vi "Launch Sample Line.vi"(8 "error in (no error)":errorcluster, 11 "cRIO-CO2 in":refnum<class "cRIO-CO2.lvclass">) -> (0 "error out":errorcluster, 3 "cRIO-CO2 out":refnum<class "cRIO-CO2.lvclass">)   [LabVIEW 2015, in "cRIO-Carbondioxide.lvlib" / "cRIO-CO2.lvlib" / "cRIO-CO2.lvclass"]
uses:
  cRIO-CO2.lvclass
  Sample Line/Sample Line.lvclass
  CO2 Actor/CO2 Actor.lvclass
  <vilib>/ActorFramework/Actor/Actor.lvclass
  cRIO-CO2.lvclass/cRIO-CO2.ctl
  cRIO-CO2 Messages/Log Message Msg/Log Message Msg.lvclass/Log Message Msg.ctl
  <vilib>/ActorFramework/Message Enqueuer/Message Enqueuer.lvclass/Message Enqueuer.ctl
  <vilib>/ActorFramework/Message Enqueuer/Enqueue.vi
  <vilib>/ActorFramework/Message Priority Queue/Priority Enqueue.vi
  <vilib>/ActorFramework/Message Enqueuer/Message Enqueuer.lvclass
  cRIO-CO2 Messages/Log Message Msg/Log Message Msg.lvclass
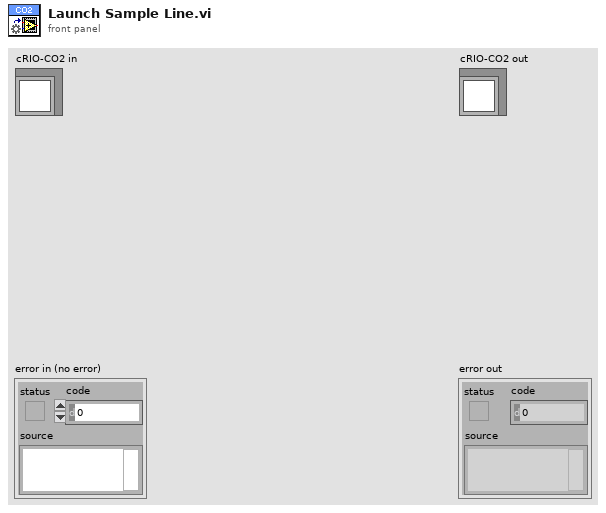
[diagram p1: front panel]
types:
  T1 = typedef "Dedicated Enqueuers.ctl" = cluster{"Freezers":cluster{"Syringe":refnum<class "Message Enqueuer.lvclass">, "Tank 1":refnum<class "Message Enqueuer.lvclass">, "Tank 2":refnum<class "Message Enqueuer.lvclass">, "Tank 3":refnum<class "Message Enqueuer.lvclass">, "Tank 4":refnum<class "Message Enqueuer.lvclass">}, "Heaters":cluster{"Syringe":refnum<class "Message Enqueuer.lvclass">, "Piston":refnum<class "Message Enqueuer.lvclass">}, "Blowers":cluster{"Tank 1":refnum<class "Message Enqueuer.lvclass">, "Tank 2":refnum<class "Message Enqueuer.lvclass">, "Tank 3":refnum<class "Message Enqueuer.lvclass">, "Tank 4":refnum<class "Message Enqueuer.lvclass">, "Syringe":refnum<class "Message Enqueuer.lvclass">}, "Sample Line":refnum<class "Message Enqueuer.lvclass">, "Storage Line":refnum<class "Message Enqueuer.lvclass">, "Transfer Line":refnum<class "Message Enqueuer.lvclass">, "Syringe Stepper":refnum<class "Message Enqueuer.lvclass">, "Syringe Line":refnum<class "Message Enqueuer.lvclass">, "Capillary Line":refnum<class "Message Enqueuer.lvclass">, "Preparation Line":refnum<class "Message Enqueuer.lvclass">, "Turbo":refnum<class "Message Enqueuer.lvclass">, "Vacuum":refnum<class "Message Enqueuer.lvclass">, "He Line":refnum<class "Message Enqueuer.lvclass">, "Cylinder":refnum<class "Message Enqueuer.lvclass">}
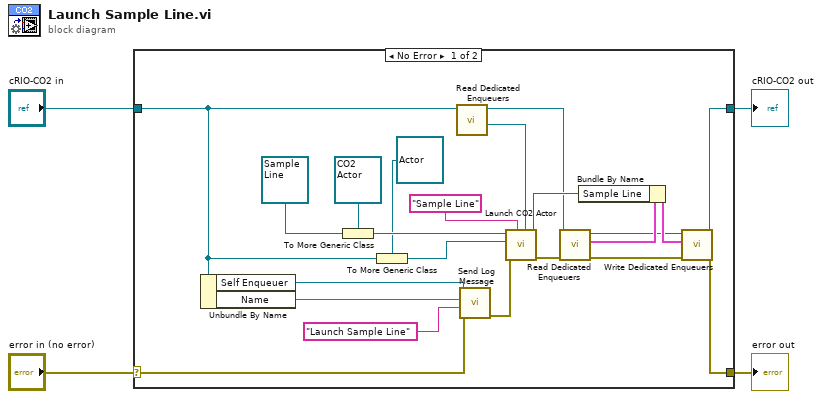
[diagram p0: block diagram]
diagram:
  n1 = case shown="No Error" "error in (no error)" {
    selector: "error in (no error)" -> [w24 w28]
    tunnel: [w14 w28] -> w3
    tunnel: [w12 w27] -> w1
    tunnel: "cRIO-CO2 in" -> [w11 w27]
    frame No Error {
      n2 = Unbundle By Name(w11) -> ("Self Enqueuer"=w7:refnum<class "Message Enqueuer.lvclass">, "Name"=w21:string)
      n3 = To More Generic Class(target class=refnum<class "CO2 Actor.lvclass"> refnum ("CO2 Actor in"), reference=refnum<class "Sample Line.lvclass"> refnum ("Sample Line.lvclass")) -> (generic class reference=w25:refnum<class "CO2 Actor.lvclass">)
      n4 = To More Generic Class(target class=refnum<class "Actor.lvclass"> refnum ("Caller Actor in"), reference=w11) -> (generic class reference=w8:refnum<class "Actor.lvclass">)
      n5 = call "Read Dedicated Enqueuers.vi"("cRIO-CO2 in"=w11) -> ("Qs.DedicatedEnQrs"=w5:refnum<queue>, "cRIO-CO2 out"=w6:refnum<class "cRIO-CO2.lvclass">)  [unwired: 7 in, 2 out]
      n6 = call "Send Log Message.vi"("error in (no error)"=w24, "String"="Launch Sample Line", "Source Name"=w21, "Message Enqueuer"=w7) -> ("error out"=w23:errorcluster)  [unwired: 6 in, 1 out]
      n7 = call "Launch CO2 Actor.vi"("DedicatedEnQrs"=w5, "Name"="Sample Line", "error in (no error)"=w23, "Caller Actor in"=w8, "CO2 Actor in"=w25) -> ("error out"=w15:errorcluster, "Caller-To-Actor Enqueuer"=w19:refnum<class "Message Enqueuer.lvclass">)  [unwired: 5 in]
      n8 = call "Read Dedicated Enqueuers.vi"("error in (no error)"=w15, "cRIO-CO2 in"=w6) -> ("error out"=w16:errorcluster, "Dedicated Enqueuers"=w18:T1, "cRIO-CO2 out"=w13:refnum<class "cRIO-CO2.lvclass">)  [unwired: 6 in, 1 out]
      n9 = Bundle By Name(cluster=w18, "Sample Line"=w19) -> (w17:T1)
      n10 = call "Write Dedicated Enqueuers.vi"("error in (no error)"=w16, "Dedicated Enqueuers"=w17, "cRIO-CO2 in"=w13) -> ("error out"=w14:errorcluster, "cRIO-CO2 out"=w12:refnum<class "cRIO-CO2.lvclass">)  [unwired: 7 in]
    }
    frame Error {
    }
  }
  "error out" <- w3
  "cRIO-CO2 out" <- w1
